vi "busy_wait.vi"(7 "caller":refnum<vi>, 8 "error in (no error)":errorcluster, 11 "configuration":T2={"dialog_text"="", "wait_s"=0.0, "inner_color"=16711680, "outer_color"=6618880, "event_registration"=refnum}) -> (0 "error out":errorcluster, 3 "dialog_selection":T1=enum."button_2")   [LabVIEW 2015, in "lv-dialog-interfaces.lvlib"]
uses:
  lv-dialog-interfaces.lvlib
  lv-dialog/api/v1/public/_controls/dialog_selection.ctl
  private/_controls/dialog_type.ctl
  private/_controls/hmi_references.ctl
  private/_controls/configuration.ctl
  lv-dialog/api/v1/v1.lvlib
panel:
  out "dialog":string
  out "busy":u16(knob) scale=0.0..20.0
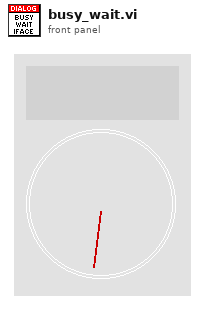
[diagram p1: front panel]
types:
  T1 = typedef "lv-dialog.lvlib/v1.lvlib/dialog_selection.ctl" = enum16{"null", "panel_closed", "button_1", "button_2", "button_3", "cancelled"}
  T2 = cluster{"dialog_text":string, "wait_s":dbl, "inner_color":u32, "outer_color":u32, "event_registration":refnum<event-registration>}
  T3 = typedef "lv-dialog-interfaces.lvlib/dialog_type.ctl" = enum16{"null", "one_button", "two_button", "three_button", "confirmation", "busy_wait", "error", "busy_wait_embed", "combo_box", "data_entry_string", "data_entry_numeric"}
  T4 = typedef "lv-dialog-interfaces.lvlib/configuration.ctl" = cluster{"dialog_text":string, "boolean_text_1":string, "boolean_text_2":string, "boolean_text_3":string, "inner_color":u32, "outer_color":u32, "wait_s":dbl, "error_status":bool, "error_source":string, "error_details":string, "string []":string[], "custom_entry":bool}
  T5 = typedef "lv-dialog-interfaces.lvlib/hmi_references.ctl" = cluster{"vi_reference":refnum<vi>, "caller":refnum<vi>, "dialog":refnum<vi>, "button_1":refnum<vi>, "button_2":refnum<vi>, "button_3":refnum<vi>, "busy":refnum<vi>, "error_glyph":refnum<vi>, "error_source":refnum<vi>, "error_text":refnum<vi>, "combo_box":refnum<vi>}
  T6 = cluster{"dialog_text":string, "boolean_text_1":string, "boolean_text_2":string}
  T7 = cluster{"dialog_text":string, "boolean_text_1":string}
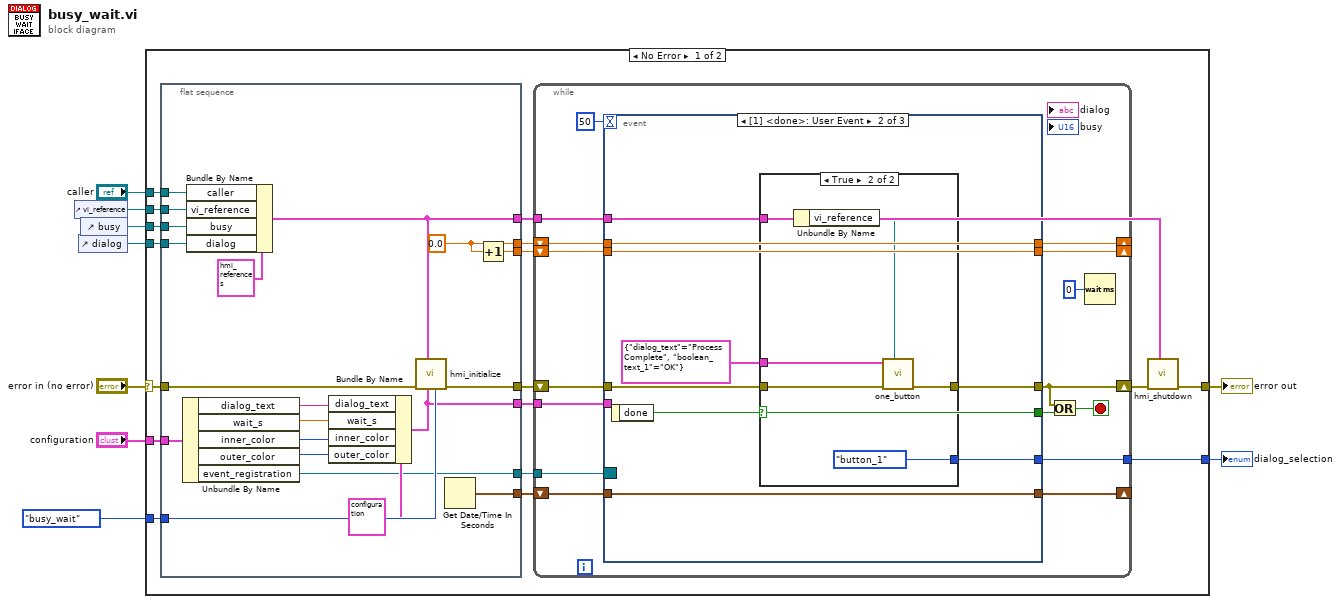
[diagram p0: block diagram]
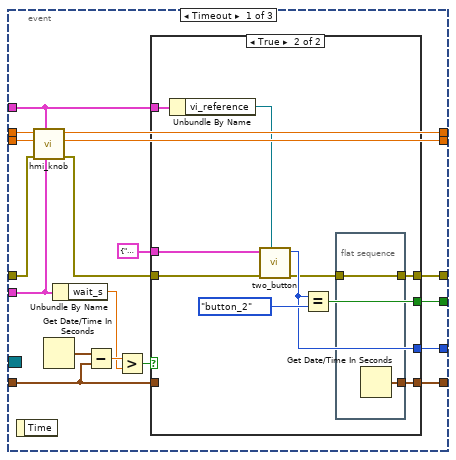
[diagram p2: hidden frame]
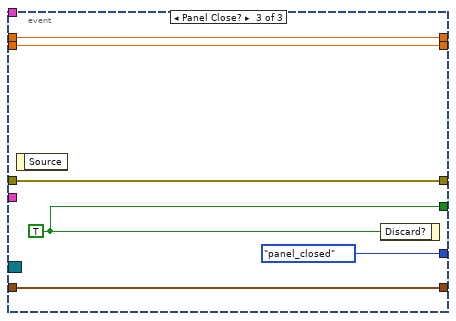
[diagram p5: hidden frame]
diagram:
  n1 = control-ref of="vi_reference"() -> (w6:refnum<vi>)
  n2 = control-ref of="dialog"() -> (w4:refnum<vi>)
  n3 = control-ref of="busy"() -> (w5:refnum<vi>)
  n4 = case shown="No Error" "error in (no error)" {
    selector: "error in (no error)" -> [w26 w117]
    tunnel: "caller" -> [w25 _]
    tunnel: "configuration" -> [w24 _]
    tunnel: [w22 w117] -> w7
    tunnel: w6 -> [w16 _]
    tunnel: w5 -> [w15 _]
    tunnel: w4 -> [w14 _]
    tunnel: dialog_type."busy_wait" ("dialog_type") -> [w13 _]
    tunnel: [w11 _] -> w1
    frame No Error {
      n5 = flat-sequence {
        tunnel: [w46] -> w21
        tunnel: [w45] -> w20
        tunnel: [w36] -> w12
        tunnel: w26 -> [w33]
        tunnel: [w32] -> w19
        tunnel: [w42] -> w18
        tunnel: w24 -> [w41]
        tunnel: [w34] -> w17
        tunnel: w25 -> [w43]
        tunnel: w16 -> [w40]
        tunnel: w15 -> [w39]
        tunnel: w14 -> [w38]
        tunnel: w13 -> [w37]
        tunnel: [w27] -> w10
        frame #0 {
          w42 = 0.0
          n6 = Unbundle By Name(w41) -> ("dialog_text"=w31:string, "wait_s"=w30:dbl, "inner_color"=w29:u32, "outer_color"=w28:u32, "event_registration"=w27:refnum<event-registration>)
          n7 = Bundle By Name(cluster=T5 {"vi_reference"=refnum, "caller"=refnum, "dialog"=refnum, "button_1"=refnum, "button_2"=refnum, "button_3"=refnum, "busy"=refnum, "error_glyph"=refnum, "error_source"=refnum, "error_text"=refnum, "combo_box"=refnum} ("references"), "caller"=w43, "vi_reference"=w40, "busy"=w39, "dialog"=w38) -> (w36:T5)
          n8 = Bundle By Name(cluster=T4 {"dialog_text"="", "boolean_text_1"="", "boolean_text_2"="", "boolean_text_3"="", "inner_color"=16711680, "outer_color"=6618880, "wait_s"=nan, "error_status"=FALSE, "error_source"="", "error_details"="", "string []"=[], "custom_entry"=FALSE} ("configuration"), "dialog_text"=w31, "wait_s"=w30, "inner_color"=w29, "outer_color"=w28) -> (w34:T4)
          n9 = call "hmi_initialize.vi"("dialog_type"=w37, "configuration"=w34, "references"=w36, "error in (no error)"=w33) -> ("error out"=w32:errorcluster)  [unwired: 7 in]
          n10 = Get Date/Time In Seconds() -> (seconds since 1Jan1904=w45:timestamp)
          n11 = Increment(x=w42) -> (x+1=w46:dbl)
        }
      }
      n12 = while {
        shift-right: [w62] -> _
        shift-left: w18 -> [w59]
        shift-right: [w61] -> _
        shift-left: w21 -> [w60]
        shift-right: [w50] -> w23
        shift-left: w19 -> [w58]
        shift-right: [w54] -> _
        shift-left: w20 -> [w55]
        tunnel: w17 -> [w53]
        tunnel: w12 -> [w49]
        tunnel: [w48] -> w11
        tunnel: w10 -> [w47]
        stop <- w51 stop-if-true
        n13 = event shown="[1] <done>: User Event" {
          selector: w47 -> [_ _ _]
          dyn-events: _ -> [_ _ _]
          timeout: 50 -> [_ _ _]
          tunnel: [w66 w103 w115] -> w62
          tunnel: [w65 w102 w114] -> w61
          tunnel: w60 -> [w75 w102 w114]
          tunnel: w59 -> [w74 w103 w115]
          tunnel: w58 -> [w80 w101 w116]
          tunnel: [w76 w100 w116] -> w50
          tunnel: [w72 w96 w113] -> w52
          tunnel: w55 -> [w67 w97 w112]
          tunnel: [w64 w97 w112] -> w54
          tunnel: w53 -> [w71 _ _]
          tunnel: w49 -> [w69 w99 _]
          tunnel: [w68 w95 dialog_selection."panel_closed" ("dialog_selection")] -> w48
          event Timeout {
            n14 = event-data() -> ()  [unwired: 1 in, 1 out]
            n15 = call "hmi_knob.vi"("configuration"=w71, "hmi_references"=w69, "error in (no error)"=w80, "value_2 in"=w75, "value_1 in"=w74) -> ("error out"=w77:errorcluster, "value_2 out"=w65:dbl, "value_1 out"=w66:dbl)  [unwired: 4 in]
            n16 = Get Date/Time In Seconds() -> (seconds since 1Jan1904=w79:timestamp)
            n17 = Unbundle By Name(w71) -> ("wait_s"=w73:dbl)
            n18 = Subtract(x=w79, y=w67) -> (x-y=w78:dbl)
            n19 = Greater?(x=w78, y=w73) -> (0:w63:bool)
            n20 = case shown="True" w63 {
              tunnel: w77 -> [w82 w90]
              tunnel: [w82 w83] -> w76
              tunnel: [_ w91] -> w72
              tunnel: T6 {"dialog_text"="Waiting process has not completed.", "boolean_text_1"="Wait", "boolean_text_2"="Continue"} -> [_ w89]
              tunnel: w69 -> [_ w88]
              tunnel: [_ w86] -> w68
              tunnel: w67 -> [w81 _]
              tunnel: [w81 w85] -> w64
              frame False {
              }
              frame True {
                n21 = Unbundle By Name(w88) -> ("vi_reference"=w87:refnum<vi>)
                n22 = call "two_button.vi"("callee"=w87, "error in (no error)"=w90, "configuration"=w89) -> ("error out"=w84:errorcluster, "dialog_selection"=w86:T1)  [unwired: 7 in]
                n23 = Equal?(x=w86, y=dialog_selection."button_2" ("x")) -> (x = y?=w91:bool)
                n24 = flat-sequence {
                  tunnel: [w94] -> w85
                  tunnel: w84 -> [w93]
                  tunnel: [w93] -> w83
                  frame #0 {
                    n25 = Get Date/Time In Seconds() -> (seconds since 1Jan1904=w94:timestamp)
                  }
                }
              }
            }
          }
          event User Event {
            n26 = event-data() -> ("done"=w96:bool)  [unwired: 1 in]
            n27 = case shown="True" w96 {
              tunnel: w101 -> [w104 w110]
              tunnel: [w104 w109] -> w100
              tunnel: w99 -> [_ w108]
              tunnel: T7 {"dialog_text"="Process Complete", "boolean_text_1"="OK"} ("configuration") -> [_ w106]
              tunnel: [_ dialog_selection."button_1" ("dialog_selection")] -> w95
              frame False {
              }
              frame True {
                n28 = Unbundle By Name(w108) -> ("vi_reference"=w107:refnum<vi>)
                n29 = call "one_button.vi"("callee"=w107, "error in (no error)"=w110, "configuration"=w106) -> ("error out"=w109:errorcluster)  [unwired: 7 in, 1 out]
              }
            }
          }
          event Panel Close? {
            w113 = TRUE
            n30 = event-data() -> ()  [unwired: 1 in, 1 out]
            n31 = event-data("Discard?"=w113) -> ()  [unwired: 1 in, 1 out]
          }
        }
        n32 = Or(x=w50, y=w52) -> (x .or. y?=w51:bool)
        n33 = Wait (ms)(milliseconds to wait=u32 0) -> ()  [unwired: 1 out]
      }
      n34 = call "hmi_shutdown.vi"("references"=w12, "error in (no error)"=w23) -> ("error out"=w22:errorcluster)  [unwired: 9 in]
    }
    frame Error {
    }
  }
  "error out" <- w7
  "dialog_selection" <- w1
